vi "mask_tdc.vi"() -> ()   [LabVIEW 2017]
panel:
  in  "error in (no error)":errorcluster
  out "error out":errorcluster
  in  "In 2":u8=132 format="%.0x"
  in  "In":u8=244 format="%.0x"
  in  "Address 2":u32=2305 format="%x"
  in  "Address":u32=2305 format="%x"
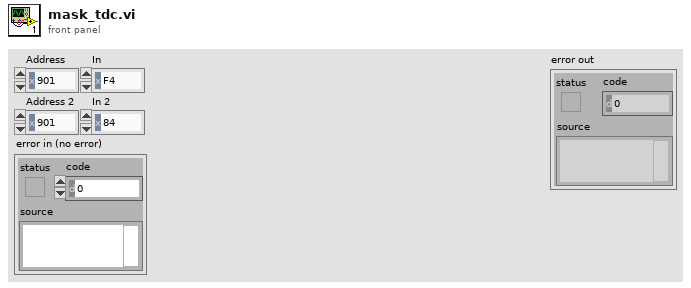
[diagram p1: front panel]
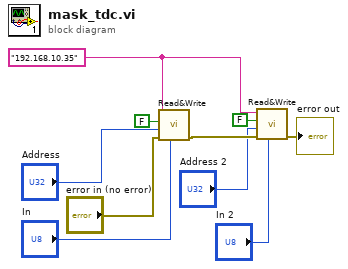
[diagram p0: block diagram]
diagram:
  w3 = "192.168.10.35" ("address")
  n1 = call "Read&Write.vi"("In"="In", "error in (no error)"="error in (no error)", "Address"="Address", "Read (TRUE)"=FALSE, "address"=w3) -> ("error out"=w10:errorcluster)  [unwired: 5 in, 1 out]
  n2 = call "Read&Write.vi"("In"="In 2", "error in (no error)"=w10, "Address"="Address 2", "Read (TRUE)"=FALSE, "address"=w3) -> ("error out"=→"error out":errorcluster)  [unwired: 5 in, 1 out]
